vi "Execute.vi"(8 "error in (no error)":errorcluster, 10 "Context in":refnum<class "Context.lvclass">, 11 "Update Command in":refnum<class "Update Command.lvclass">) -> (0 "error out":errorcluster, 2 "Context out":refnum<class "Context.lvclass">, 3 "Update Command out":refnum<class "Update Command.lvclass">)   [LabVIEW 2016, in "Update Command.lvclass"]
uses:
  Update Command.lvclass
  Context/Context.lvclass
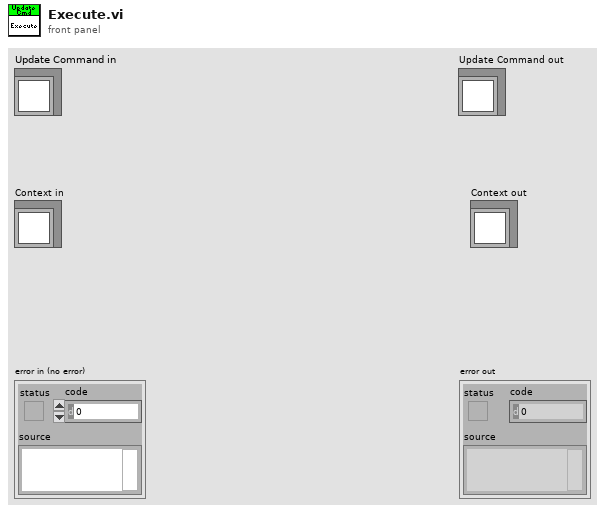
[diagram p1: front panel]
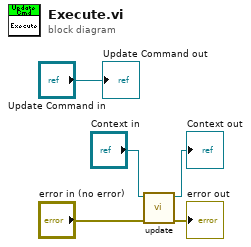
[diagram p0: block diagram]
diagram:
  n1 = call "update.vi"("error in (no error)"="error in (no error)", "Context in"="Context in") -> ("error out"=→"error out":errorcluster, "Context out"=→"Context out":refnum<class "Context.lvclass">)  [unwired: 8 in]
  "Update Command out" <- "Update Command in"
